vi "ExternalGetParam.vi"(0 "reference":refnum<class "ClassNode.lvclass">, 1 "setParameter":T2, 5 "error in (no error)":errorcluster) -> (14 "reference out":refnum<class "ClassNode.lvclass">, 15 "string":string, 16 "position":T1 {"y" format="%.2f"; "x" format="%.2f"}, 17 "Boolean":bool, 18 "Path":path, 19 "error out":errorcluster)   [LabVIEW 2016, in "ClassNode.lvclass"]
doc: "Sets parameter externaly.\nPossible to set Name,Attrib,Methods and Position"
uses:
  <resource>/Framework/Providers/Open_GDS/UML/ClassNode_class/ClassNode.lvclass
  C:/Program Files (x86)/National Instruments/LabVIEW 2016/resource/Framework/Providers/Open_GDS/UML/RectangularNode_class/RectangularNode.lvclass
  <resource>/Framework/Providers/Open_GDS/UML/ClassNode_class/ExternalSetTypes.ctl
  <resource>/Framework/Providers/Open_GDS/UML/General/Point/Point Point2D.ctl
  <resource>/Framework/Providers/Open_GDS/UML/MultiLineString_class/MultiLineString.lvclass
  <resource>/Framework/Providers/Open_GDS/UML/RectangularNode_class/RectangularNode.lvclass
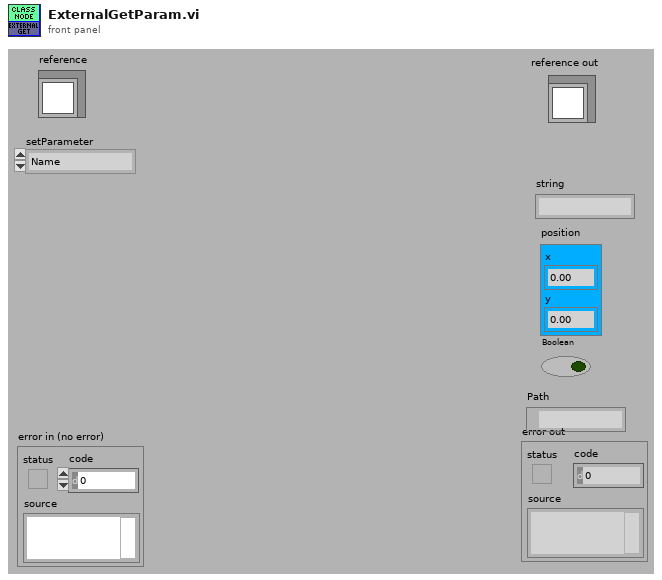
[diagram p1: front panel]
types:
  T1 = typedef "Point Point2D.ctl" = cluster{"x":dbl, "y":dbl}
  T2 = typedef "ClassNode.lvclass/ExternalSetTypes.ctl" = enum16{"Name", "Attributes", "Methods", "Position", "ShowMethods", "ShowAttributes", "ClassPath"}
  T3 = typedef "ClassNode.lvclass/ObjectAttributes.ctl" = cluster{"midHeight":dbl, "botHeight":dbl, "name":refnum<class "MultiLineString.lvclass">, "attributes":refnum<class "MultiLineString.lvclass">, "methods":refnum<class "MultiLineString.lvclass">, "DEFAULT_COMPARTMENT_HEIGHT":i32, "DEFAULT_WIDTH":i32, "DEFAULT_HEIGHT":i32, "showMethods":bool, "showAttributes":bool, "ClassPath":path}
  T4 = typedef "RectangularNode.lvclass/ObjectAttributes.ctl" = cluster{"bounds":T5}
  T5 = typedef "Rectangle Rectangle2D.ctl" = cluster{"x":dbl, "y":dbl, "width":dbl, "height":dbl}
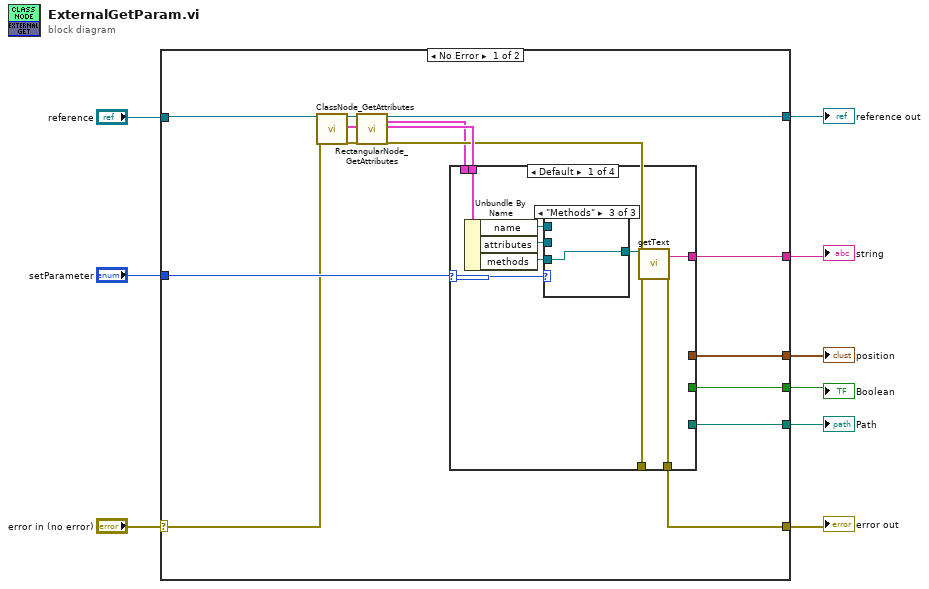
[diagram p0: block diagram]
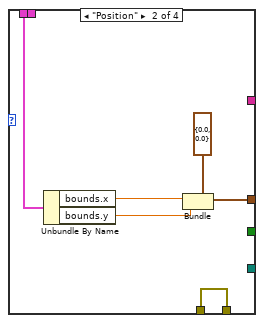
[diagram p4: hidden frame]
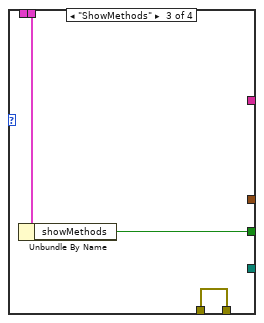
[diagram p5: hidden frame]
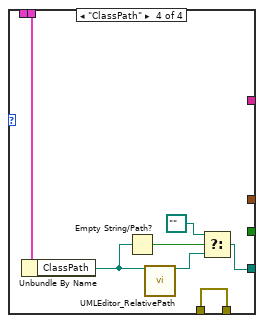
[diagram p6: hidden frame]
diagram:
  n1 = case shown="No Error" "error in (no error)" {
    selector: "error in (no error)" -> [w21 w52]
    tunnel: "reference" -> [w23 w53]
    tunnel: [w20 w52] -> w7
    tunnel: [w11 w53] -> w6
    tunnel: "setParameter" -> [w22 _]
    tunnel: [w19 _] -> w3
    tunnel: [w18 _] -> w4
    tunnel: [w17 _] -> w2
    tunnel: [w16 _] -> w1
    frame No Error {
      n2 = call <resource>:"ClassNode_GetAttributes.vi"("reference in"=w23, "error in (no error)"=w21) -> ("reference out"=w14:refnum<class "ClassNode.lvclass">, "Data"=w15:T3, "error out"=w13:errorcluster)  [unwired: 1 in, 14 out]
      n3 = call <resource>:"RectangularNode_GetAttributes.vi"("reference in"=w14, "error in (no error)"=w13) -> ("reference out"=w11:refnum<class "ClassNode.lvclass">, "Data"=w10:T4, "error out"=w12:errorcluster)  [unwired: 14 in, 1 out]
      n4 = case shown="Default" w22 {
        selector: w22 -> [w32 _ _ _]
        tunnel: w12 -> [w31 w41 w44 w51]
        tunnel: [w30 w41 w44 w51] -> w20
        tunnel: [_ w37 _ _] -> w19
        tunnel: [_ _ w43 _] -> w18
        tunnel: [w25 _ _ _] -> w17
        tunnel: [_ _ _ w47] -> w16
        tunnel: w15 -> [w24 _ w42 w45]
        tunnel: w10 -> [_ w36 _ _]
        frame Default {
          n5 = Unbundle By Name(w24) -> ("name"=w29:refnum<class "MultiLineString.lvclass">, "attributes"=w27:refnum<class "MultiLineString.lvclass">, "methods"=w26:refnum<class "MultiLineString.lvclass">)
          n6 = case shown="\"Methods\"" w32 {
            tunnel: w29 -> [w33 _ _]
            tunnel: [w33 w34 w35] -> w28
            tunnel: w27 -> [_ w34 _]
            tunnel: w26 -> [_ _ w35]
            frame "Name", Default {
            }
            frame "Attributes" {
            }
            frame "Methods" {
            }
          }
          n7 = call-dynamic "getText.vi"("reference"=w28, "error in (no error)"=w31) -> ("text"=w25:string, "error out"=w30:errorcluster)  [unwired: 16 out]
        }
        frame "Position" {
          n8 = Unbundle By Name(w36) -> ("bounds.x"=w39:dbl, "bounds.y"=w38:dbl)
          n9 = Bundle(cluster=T1 {"x"=0.0, "y"=0.0} ("position"), "x"=w39, "y"=w38) -> (w37:T1)
        }
        frame "ShowMethods" {
          n10 = Unbundle By Name(w42) -> ("showMethods"=w43:bool)
        }
        frame "ClassPath" {
          n11 = Unbundle By Name(w45) -> ("ClassPath"=w50:path)
          n12 = Empty String/Path?(string/path=w50) -> (empty?=w49:bool)
          n13 = call <resource>:"UMLEditor_RelativePath.vi"("Path In"=w50) -> ("ConvertToAbsolutePath(If possible)"=w48:path)  [unwired: 1 in, 17 out]
          n14 = Select(t=path "", s=w49, f=w48) -> (s? t:f=w47:path)
        }
      }
    }
    frame Error {
    }
  }
  "reference out" <- w6
  "error out" <- w7
  "position" <- w3
  "string" <- w2
  "Boolean" <- w4
  "Path" <- w1
